vi "setOutputWaveform.vi"(7 "Channel":string="0", 8 "error in (no error)":errorcluster, 10 "Type":T1, 11 "FgenNiPxi in":refnum<class "ArbNi.lvclass">) -> (0 "error out":errorcluster, 3 "FgenNiPxi out":refnum<class "ArbNi.lvclass">)   [LabVIEW 2023, in "ArbNi.lvclass"]
doc: "<b>Author:</b> Wolfgang\n<b>Description:</b> Set waveform type per channel"
uses:
  ArbNi.lvclass
  Data/arbWaveformType.ctl
  ArbNi.lvclass/ArbNi.ctl
  <instrlib>/niFgen/niFgen.llb/niFgen Waveform Type.ctl
  Arb.lvclass
  sweArb.lvlib
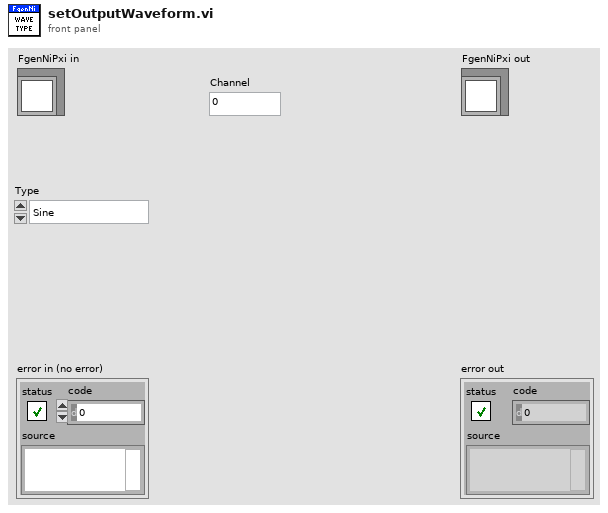
[diagram p1: front panel]
types:
  T1 = typedef "sweArb.lvlib/arbWaveformType.ctl" = enum16{"Sine", "Square", "Triangle", "DC", "Noise", "Arb"}
  T2 = typedef "niFgen Waveform Type.ctl" = i32
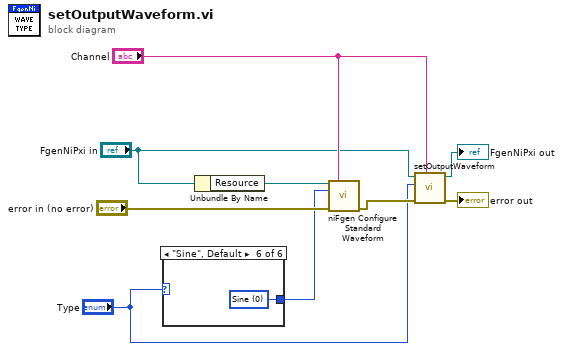
[diagram p0: block diagram]
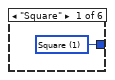
[diagram p2: hidden frame]
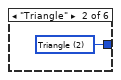
[diagram p3: hidden frame]
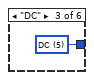
[diagram p4: hidden frame]
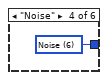
[diagram p5: hidden frame]
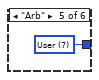
[diagram p6: hidden frame]
diagram:
  n1 = case shown="\"Sine\", Default" "Type" {
    tunnel: [w10 w11 w12 w13 w14 w15] -> w5
    frame "Square" {
      w10 = T2 1 items=["Sine", "Square", "Triangle", "Ramp Up", "Ramp Down", "DC", "Noise", "User"] ("Waveform")
    }
    frame "Triangle" {
      w11 = T2 2 items=["Sine", "Square", "Triangle", "Ramp Up", "Ramp Down", "DC", "Noise", "User"] ("Waveform")
    }
    frame "DC" {
      w12 = T2 5 items=["Sine", "Square", "Triangle", "Ramp Up", "Ramp Down", "DC", "Noise", "User"] ("Waveform")
    }
    frame "Noise" {
      w13 = T2 6 items=["Sine", "Square", "Triangle", "Ramp Up", "Ramp Down", "DC", "Noise", "User"] ("Waveform")
    }
    frame "Arb" {
      w14 = T2 7 items=["Sine", "Square", "Triangle", "Ramp Up", "Ramp Down", "DC", "Noise", "User"] ("Waveform")
    }
    frame "Sine", Default {
      w15 = T2 0 items=["Sine", "Square", "Triangle", "Ramp Up", "Ramp Down", "DC", "Noise", "User"] ("Waveform")
    }
  }
  n2 = Unbundle By Name("FgenNiPxi in") -> ("Resource"=w8:refnum<k15>)
  n3 = call <instrlib>:"niFgen Configure Standard Waveform.vi"("Instrument Handle"=w8, "Channel Name"="Channel", "Waveform"=w5, "error in (no error)"="error in (no error)") -> ("error out"=w4:errorcluster)  [unwired: 10 in, 1 out]
  n4 = call-parent "setOutputWaveform.vi"("Channel"="Channel", "error in (no error)"=w4, "Type"="Type", "Fgen in"="FgenNiPxi in") -> ("error out"=→"error out":errorcluster, "Fgen out"=→"FgenNiPxi out":refnum<class "ArbNi.lvclass">)  [unwired: 6 in]
